vi "Configure Multi Data Save.vi"(0 "VISA resource name":refnum<visa-resource-name>, 1 "Batch Group Number  [/BT] (1)":i32=1 min=1 max=12, 2 "File Header Characters (\"\")":string, 3 "Data File Name Structure (0: Date)":u16(ring) items=["Date", "Serial", "Batch"], 4 "Data File Name Identified Strings (\"\")":string, 5 "error in (no error)":errorcluster) -> (14 "VISA resource name out":refnum<visa-resource-name>, 19 "error out":errorcluster)   [LabVIEW 2020, in "Yokogawa GX Series.lvlib"]
doc: "Set data save (/BT Option)\n\nCommand: SMltFileHead\n SMltFileName"
uses:
  <instrlib>/Yokogawa GX Series/Yokogawa GX Series.lvlib
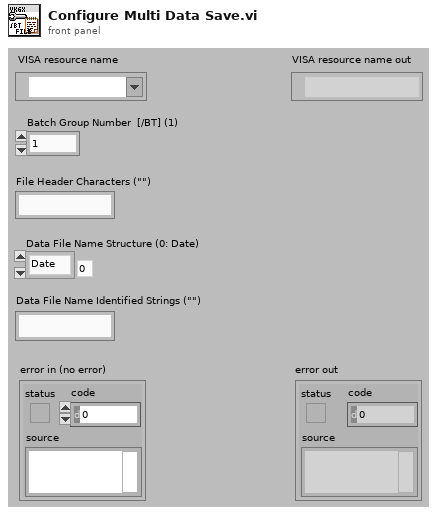
[diagram p1: front panel]
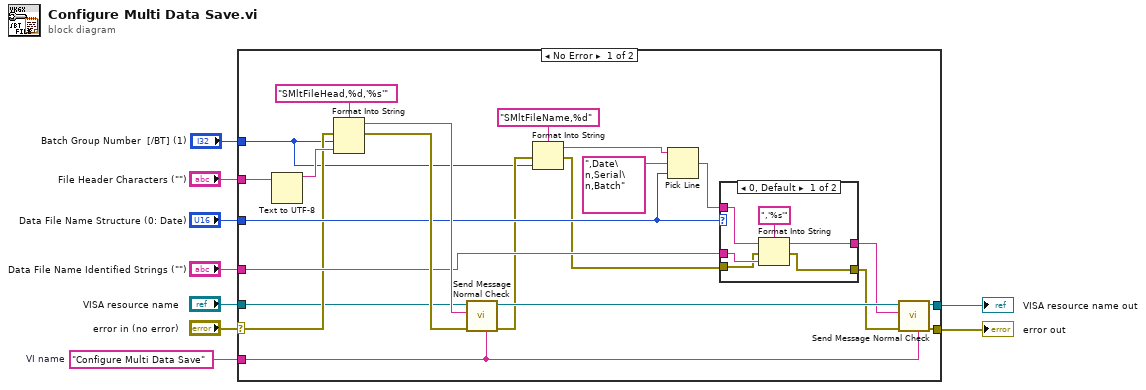
[diagram p0: block diagram]
diagram:
  w3 = "Configure Multi Data Save"  # VI name
  n1 = case shown="No Error" "error in (no error)" {
    selector: "error in (no error)" -> [w18 w40]
    tunnel: "VISA resource name" -> [w17 w41]
    tunnel: "File Header Characters (\"\")" -> [w20 _]
    tunnel: "Data File Name Structure (0: Date)" -> [w28 _]
    tunnel: "Data File Name Identified Strings (\"\")" -> [w26 _]
    tunnel: [w16 w41] -> w5
    tunnel: [w15 w40] -> w4
    tunnel: w3 -> [w22 _]
    tunnel: "Batch Group Number  [/BT] (1)" -> [w12 _]
    frame No Error {
      n2 = Text to UTF-8(11:w20) -> (3:w19:string)  [unwired: 2 in, 1 out]
      n3 = Format Into String(format string="SMltFileHead,%d,'%s'", error in=w18, w12, w19) -> (resulting string=w29:string, error out=w30:errorcluster)  [unwired: 1 in]
      n4 = call <instrlib>:"Send Message Normal Check.vi"("Source (\"\")"=w22, "error in (no error)"=w30, "Send Message (\"\")"=w29, "VISA resource name"=w17) -> ("error out"=w13:errorcluster, "VISA resource name out"=w25:refnum<visa-resource-name>)  [unwired: 2 in, 4 out]
      n5 = Format Into String(format string="SMltFileName,%d", error in=w13, w12) -> (resulting string=w11:string, error out=w10:errorcluster)  [unwired: 1 in]
      n6 = Pick Line(string ("")=w11, multi-line string=",Date\n,Serial\n,Batch", line index=w28) -> (output string=w27:string)
      n7 = case shown="0, Default" w28 {
        tunnel: w27 -> [w37 w39]
        tunnel: w26 -> [w35 _]
        tunnel: [w34 w38] -> w24
        tunnel: [w33 w39] -> w23
        tunnel: w10 -> [w32 w38]
        frame 0, Default {
          n8 = Format Into String(format string=",'%s'", initial string=w37, error in=w32, w35) -> (resulting string=w33:string, error out=w34:errorcluster)
        }
        frame 2 {
        }
      }
      n9 = call <instrlib>:"Send Message Normal Check.vi"("Source (\"\")"=w22, "error in (no error)"=w24, "Send Message (\"\")"=w23, "VISA resource name"=w25) -> ("error out"=w15:errorcluster, "VISA resource name out"=w16:refnum<visa-resource-name>)  [unwired: 2 in, 4 out]
    }
    frame Error {
    }
  }
  "error out" <- w4
  "VISA resource name out" <- w5
